vi "Meas Main.vi"(8 "error in":errorcluster, 11 "session in":variant) -> (0 "error out":errorcluster, 3 "session out":variant)   [LabVIEW 2013]
uses:
  Meas Session.ctl
  adc/ADC Session.ctl
  drivers/niScope/niScope Session.ctl
  drivers/niScope/niScope Virtual Channel Config.ctl
  drivers/niScope/niScope Virtual Channel Mode.ctl
  drivers/niScope/niScope Virtual Channel Input Z.ctl
  drivers/niScope/niScope Virtual Channel Coupling.ctl
  drivers/niScope/niScope Type.ctl
  drivers/niScope/niScope Digitizing Process Options.ctl
  drivers/niScope/niScope Data Packet.ctl
  drivers/niScope/niScope Trigger Setup.ctl
  <instrlib>/niScope/Controls/niScope trigger coupling.ctl
  <instrlib>/niScope/Controls/niScope trigger slope.ctl
  drivers/DMM/3458A Digitizer Session.ctl
  drivers/DMM/3458A Virtual Channel Config.ctl
  drivers/Counter/Counter Session.ctl
  drivers/Counter/Counter Type.ctl
  drivers/AWG/AWG Session.ctl
  drivers/AWG/AWG Type.ctl
  drivers/DMM/3458A Sync Mode.ctl
  drivers/DMM/3458A Idn Mode.ctl
  drivers/DMM/3458A Digitizing Low Levels/Configure/Sampling Mode.ctl
  drivers/DMM/3458A Digitizing Process Options.ctl
  drivers/DMM/3458A Data Packet.ctl
  drivers/DMM/3458A Aux Record Data.ctl
  drivers/DMM/3458A Digitizing Low Levels/Configure/Level Setup.ctl
  drivers/DMM/3458A Digitizing Low Levels/Configure/First Sample Trigger.ctl
  drivers/dsdll/DSDLL Session.ctl
  drivers/dsdll/dsdll.lvlibp/dsdll_instance.ctl
  drivers/dsdll/dsdll.lvlibp/dsdll_device_record.ctl
  drivers/dsdll/DSDLL Process Config.ctl
  drivers/dsdll/DSDLL Data Packet.ctl
  adc/ADC Type.ctl
  drivers/simulated_adc/SimAdc Config.ctl
  drivers/simulated_adc/SimAdc Channel Cfg.ctl
  adc/ADC On Close Action.ctl
  Meas Sequence Item.ctl
  Meas Sampling Configuration.ctl
  adc/ADC Trig Config.ctl
  adc/ADC Trig Mode Source.ctl
  adc/ADC Trig Coupling.ctl
  adc/ADC Trig Slope.ctl
  processing/QWTB/Meas Proc QWTB Algorithm Parameter Data.ctl
  Meas Sequence Configuration.ctl
  Meas Range Mode.ctl
  Meas Sampling Rate Mode.ctl
  octave/golpi/mpc/golpi_session_ref.ctl
  processing/Meas Process Config.ctl
  processing/Meas Process Mode.ctl
  processing/Meas Process Raw Config.ctl
  processing/Meas Process Raw Result Mode.ctl
  processing/QWTB/Meas Proc QWTB Setup.ctl
  processing/QWTB/Meas Proc QWTB Uncertainty Mode.ctl
  processing/QWTB/Meas Proc QWTB Multicore Setup.ctl
  processing/QWTB/Meas Proc QWTB Multicore Type.ctl
  Corrections/Corr Setup.ctl
  Corrections/Corr Tranducer Item.ctl
  Corrections/Corr Digitizers.ctl
  Assist/Assist Panel Setup.ctl
  varilib/SGUI Assign Multiple Strings With Tags By Label.vi
  drivers/niScope/niScope Virtual Digitizer.lvlib
  drivers/DMM/3458A Virtual Digitizer.lvlib
  drivers/Counter/Counter.lvlib
  drivers/AWG/AWG.lvlib
  drivers/DMM/3458A Digitizing Low Levels/3458A Digitizing Low Levels.lvlib
  varilib/varilib.lvlib
  drivers/dsdll/DSDLL Virtual Digitizer.lvlib
  drivers/dsdll/dsdll.lvlibp
  octave/golpi/mpc/GOLPI Multi Process.lvlib
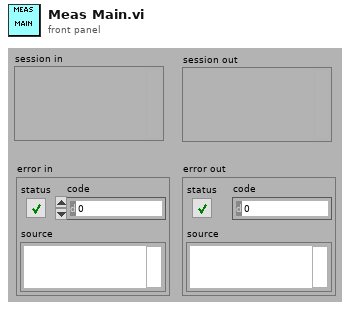
[diagram p1: front panel]
types:
  T1 = typedef "Meas Session.ctl" = cluster{"adc":T2, "sequence":T35[], "sequence setup":T42, "golpi":T45, "processing setup":T46, "corrections":T54, "assist cfg":T57}
  T2 = typedef "ADC Session.ctl" = cluster{"niScope":T3, "3458A":T13, "dsdll":T27, "type":T31, "channel idn str":string[], "aux instr idn str":string[], "modified?":bool, "simadc":T32, "force rst?":bool, "exit mode":T34, "exit dly":dbl, "exit tmr":timestamp, "busy?":bool, "accessed?":bool}
  T3 = typedef "niScope Virtual Digitizer.lvlib/niScope Session.ctl" = cluster{"channel cfg":T4[], "sessions":refnum<k20>[], "multi cards":bool, "channels":i32, "type":T8, "memory [B/chn]":i32, "ext. clock [Hz]":dbl, "samples count":i64, "use streaming":bool, "proc setup":T9, "sample width [B]":i32, "ranges [V]":dbl[], "trigger setup":T10, "fs [Hz]":dbl, "bitres [bit]":i32}
  T4 = typedef "niScope Virtual Digitizer.lvlib/niScope Virtual Channel Config.ctl" = cluster{"Address":refnum<k15>, "Channel":i32, "Mode":T5, "Input Z":T6, "Coupling":T7, "Range [Vpk]":dbl, "btn clr":bool, "btn up":bool, "btn down":bool}
  T5 = typedef "niScope Virtual Digitizer.lvlib/niScope Virtual Channel Mode.ctl" = enum16{"Single ended", "Unbal. differential", "Differential"}
  T6 = typedef "niScope Virtual Digitizer.lvlib/niScope Virtual Channel Input Z.ctl" = enum16{"1 MOhm", "50 Ohm"}
  T7 = typedef "niScope Virtual Digitizer.lvlib/niScope Virtual Channel Coupling.ctl" = enum16{"AC", "DC", "GND"}
  T8 = typedef "niScope Virtual Digitizer.lvlib/niScope Type.ctl" = enum16{"n/a", "5922"}
  T9 = typedef "niScope Virtual Digitizer.lvlib/niScope Digitizing Process Options.ctl" = cluster{"packet size [smpl]":i64, "current timeout [s]":dbl, "blk2blk timeout [s]":dbl, "event time":timestamp, "temp sampl T [s]":dbl, "data queue":refnum<queue>, "stop notifier":refnum<notifier>, "proc ref":refnum<vi>}
  T10 = typedef "niScope Virtual Digitizer.lvlib/niScope Trigger Setup.ctl" = cluster{"coupling":T11, "level [V]":dbl, "slope":T12, "mode":enum16{"Immediate", "External", "Level"}}
  T11 = typedef "niScope trigger coupling.ctl" = u16
  T12 = typedef "niScope trigger slope.ctl" = i32
  T13 = typedef "3458A Virtual Digitizer.lvlib/3458A Digitizer Session.ctl" = cluster{"channels":T14[], "sync unit":T15, "awg unit":T17, "sync mode":T19, "streaming mode":bool, "idn mode":T20, "sampling mode":T21, "Ts [s]":dbl, "sample memory [B]":i32, "proc setup":T22, "sample size [B]":i32, "sample count":i32, "aux data":T24, "ranges [V]":dbl[], "aperture [s]":dbl, "LEVEL trigger":T25, "trigger mode":T26, "measure temp.?":bool, "disp mesages":string[], "shared bus?":bool, "disable display?":bool}
  T14 = typedef "3458A Virtual Digitizer.lvlib/3458A Virtual Channel Config.ctl" = cluster{"VISA":refnum<visa-resource-name>, "Range [Vpk]":dbl, "btn clr":bool, "btn up":bool, "btn down":bool}
  T15 = typedef "Counter.lvlib/Counter Session.ctl" = cluster{"VISA":refnum<visa-resource-name>, "type":T16}
  T16 = typedef "Counter.lvlib/Counter Type.ctl" = enum16{"Picotest U6200A", "dummy"}
  T17 = typedef "AWG.lvlib/AWG Session.ctl" = cluster{"type":T18, "VISA":refnum<visa-resource-name>, "enable 10MHz ref":bool}
  T18 = typedef "AWG.lvlib/AWG Type.ctl" = enum16{"Agilent 331xxA to 332xxA", "Agilent 335xxA to 336xxA", "dummy"}
  T19 = typedef "3458A Virtual Digitizer.lvlib/3458A Sync Mode.ctl" = enum16{"MASTER-SLAVE, MASTER clocked by TIMER", "MASTER-SLAVE, MASTER clocked by AWG", "ALL clocked by AWG", "MASTER-SLAVE, ALL clocked by TIMER", "ALL clocked by AWG with DFLL"}
  T20 = typedef "3458A Virtual Digitizer.lvlib/3458A Idn Mode.ctl" = enum16{"Auto", "Sequential (chn A, chn B, ...)", "From calibration string"}
  T21 = typedef "3458A Virtual Digitizer.lvlib/3458A Digitizing Low Levels.lvlib/Sampling Mode.ctl" = enum16{"DCV", "DSDC", "DSAC"}
  T22 = typedef "3458A Virtual Digitizer.lvlib/3458A Digitizing Process Options.ctl" = cluster{"channel id":i32, "packet size [smpl]":i32, "current timeout [s]":dbl, "blk2blk timeout [s]":dbl, "event time":timestamp, "stop notifier":refnum<notifier>, "data queues":refnum<queue>[], "proc refs":refnum<vi>[], "bus semaphore":T23}
  T23 = typedef "Semaphore RefNum" = refnum<k1>
  T24 = typedef "3458A Virtual Digitizer.lvlib/3458A Aux Record Data.ctl" = cluster{"channel id":i32, "valid?":bool[], "gain [V]":dbl[], "timestamp [s]":dbl[], "Ts [s]":dbl, "abs timestamp":timestamp, "t [deg C]":dbl[]}
  T25 = typedef "3458A Virtual Digitizer.lvlib/3458A Digitizing Low Levels.lvlib/Level Setup.ctl" = cluster{"edge":enum16{"POS", "NEG"}, "level [V]":dbl, "coupling":enum16{"DC", "AC"}}
  T26 = typedef "3458A Virtual Digitizer.lvlib/3458A Digitizing Low Levels.lvlib/First Sample Trigger.ctl" = enum16{"AUTO", "EXT", "SYN", "SGL", "HOLD", "LEVEL"}
  T27 = typedef "DSDLL Virtual Digitizer.lvlib/DSDLL Session.ctl" = cluster{"dsdll":T28, "channels":i32, "device id":i32, "channel idns":string[], "proc setup":T30, "samples count":i32, "fs [Hz]":dbl}
  T28 = typedef "dsdll.lvlibp/dsdll_instance.ctl" = cluster{"dsdll path":path, "dsdll handle":u8[], "output devices":T29[], "capture devices":T29[]}
  T29 = typedef "dsdll.lvlibp/dsdll_device_record.ctl" = cluster{"guid":u8[], "name":string}
  T30 = typedef "DSDLL Virtual Digitizer.lvlib/DSDLL Process Config.ctl" = cluster{"packet size [smpl]":i32, "current timeout [s]":dbl, "blk2blk timeout [s]":dbl, "event time":timestamp, "data queue":refnum<queue>, "stop notifier":refnum<notifier>, "proc ref":refnum<vi>}
  T31 = typedef "ADC Type.ctl" = enum16{"niScope", "3458A", "DirectSound DLL", "dummy"}
  T32 = typedef "SimAdc Config.ctl" = cluster{"channels":T33[], "range [V]":dbl, "Ts step [s]":dbl, "time [s]":dbl, "fs [Hz]":dbl, "count":i64, "smpl offset":i64, "set count":i64, "bit res":i32}
  T33 = typedef "SimAdc Channel Cfg.ctl" = cluster{"harmonics":dbl[][], "btn clear":bool, "noise":dbl, "fundamental [Hz]":dbl}
  T34 = typedef "ADC On Close Action.ctl" = enum16{"Immediate reset", "Delayed reset"}
  T35 = typedef "Meas Sequence Item.ctl" = cluster{"config":T36, "data file path":path, "header file path":path, "group id":i32, "average id":i32, "group done?":bool, "adc modified?":bool, "source modified?":bool, "progress [%]":dbl, "groups cnt":i32, "average cnt":i32, "data file relative path":string, "meas root path":path, "calculate?":bool}
  T36 = typedef "Meas Sampling Configuration.ctl" = cluster{"fs [Hz]":dbl, "count [smpl]":i64, "aperture [s]":dbl, "trigger":T37, "ranges [Vpk]":dbl[], "QWTB parameters":T41[]}
  T37 = typedef "ADC Trig Config.ctl" = cluster{"source":T38, "level [V]":dbl, "coupling":T39, "slope":T40}
  T38 = typedef "ADC Trig Mode Source.ctl" = enum16{"Immediate", "External", "Level"}
  T39 = typedef "ADC Trig Coupling.ctl" = enum16{"DC", "AC"}
  T40 = typedef "ADC Trig Slope.ctl" = enum16{"POS", "NEG"}
  T41 = typedef "Meas Proc QWTB Algorithm Parameter Data.ctl" = cluster{"name":string, "numerics":dbl[], "strings":string[]}
  T42 = typedef "Meas Sequence Configuration.ctl" = cluster{"group setups":T36[], "average cycles":i32, "range mode":T43, "fs mode":T44, "rng even":dbl, "rng odd":dbl, "folder":path, "name base":string, "meas id":i32, "settle [s]":dbl}
  T43 = typedef "Meas Range Mode.ctl" = enum16{"Keep defaults", "Set All channels", "Set Odd and Even channels"}
  T44 = typedef "Meas Sampling Rate Mode.ctl" = enum16{"Frequency", "Period"}
  T45 = typedef "GOLPI Multi Process.lvlib/golpi_session_ref.ctl" = refnum<vi>
  T46 = typedef "Meas Process Config.ctl" = cluster{"mode":T47, "call after avgs?":bool, "calculate?":bool, "raw mode":T48, "QWTB":T50}
  T47 = typedef "Meas Process Mode.ctl" = enum16{"Raw", "QWTB"}
  T48 = typedef "Meas Process Raw Config.ctl" = cluster{"command":string, "result mode":T49, "res variable":string}
  T49 = typedef "Meas Process Raw Result Mode.ctl" = enum16{"Display console output (only Octave)", "Display string variable", "Display result file %respath%"}
  T50 = typedef "Meas Proc QWTB Setup.ctl" = cluster{"QWTB path":path, "alg filter path":string, "alg ids":string[], "alg parameters":string[], "parsed parameters":T41[], "selected alg id":string, "selected unc mode":T51, "qwtb mcc":i32, "qwtb timeout":i32, "qwtb covg":dbl, "qwtb ofs":i64, "qwtb lim data":i64, "multicore":T52, "unc once?":bool}
  T51 = typedef "Meas Proc QWTB Uncertainty Mode.ctl" = enum16{"None", "GUF", "Monte Carlo"}
  T52 = typedef "Meas Proc QWTB Multicore Setup.ctl" = cluster{"jobs folder":path, "cores":i32, "max jobs":i32, "mode":T53}
  T53 = typedef "Meas Proc QWTB Multicore Type.ctl" = enum16{"Singlecore", "Multicore", "Multistation"}
  T54 = typedef "Corr Setup.ctl" = cluster{"transducers":cluster{"channels":T55[], "last path":path}, "digitizer":T56}
  T55 = typedef "Corr Tranducer Item.ctl" = cluster{"Path":path, "Ratio:":string, "Name:":string, "btn rem":bool, "btn up":bool, "btn down":bool, "s.n.:":string, "btn open":bool, "ratio o/i":dbl, "chn hi":u16, "chn lo":u16, "Phase index":i32}
  T56 = typedef "Corr Digitizers.ctl" = cluster{"last path":path, "channel paths":path[], "channel idns":string[], "correction name":string, "channel names":string[], "folders to copy":path[], "channel valid":bool[], "correction path":path, "correction rel path":string, "rel folders to copy":string[]}
  T57 = typedef "Assist Panel Setup.ctl" = cluster{"P":i32, "Q":i32, "rel shift":dbl, "ref freq":dbl, "min fs":dbl, "max fs tol":dbl, "min int":dbl, "max int":dbl, "max err":dbl, "max timeout":dbl}
  T58 = typedef "GOLPI Multi Process.lvlib/golpi_session.ctl" = cluster{"GOLPI ref":T59, "idn str":string, "octave path":path, "work path":path, "start timeout [ms]":u32, "clr cache":bool, "console":bool, "binary":bool, "semaphore":T23, "initial command":string, "exit command":string, "matlab":bool}
  T59 = typedef "GOLPI Library.lvlibp/GOLPI reference Type Def.ctl" = cluster{"pipe handle":T60, "fast read timeout [ms]":u32, "fast read settle time [ms]":u32, "fast read to multiple [ms]":u32, "max elements per input line":u32, "slow read timeout [ms]":u32, "stdin double format specifier":string, "max elements per stdout output column":u32, "console mode bitstream":bool, "bitstream first read timeout [ms]":u32, "bitstream read timeout [ms]":u32, "struct transfer possible":bool, "matlab mode":bool}
  T60 = typedef "GOLPI Library.lvlibp/LV Process library.lvlib/Pipe Handle.ctl" = cluster{"lv_proc.dll file path":path, "process instance handle":u32[], "debug mode":bool, "debug data":cluster{"time":timestamp, "stdin":bool, "data":string}[]}
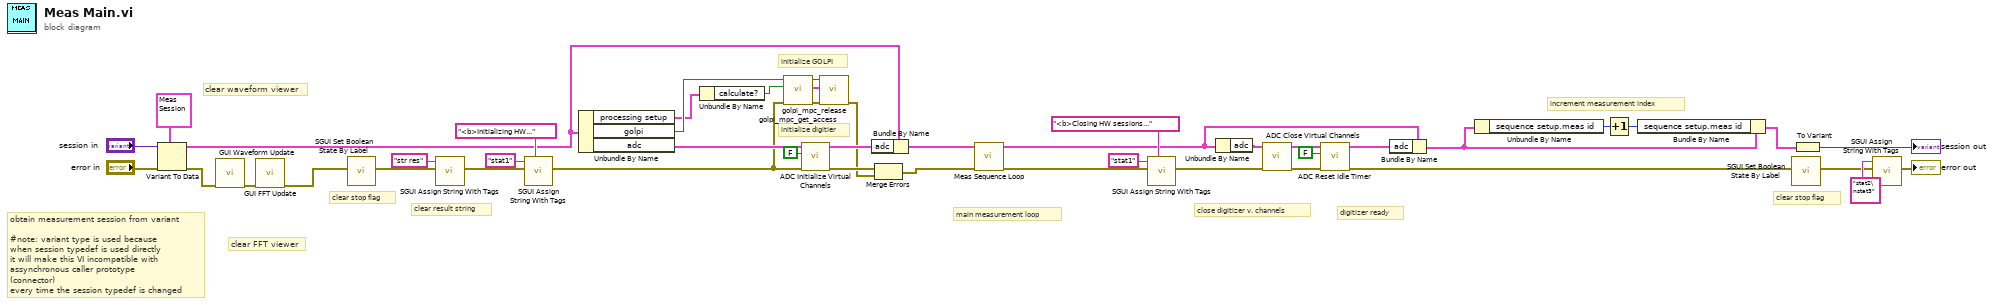
[diagram p0: block diagram]
diagram:
  # "clear FFT viewer"
  # "main measurement loop"
  # "digitizer ready"
  # "close digitizer v. channels"
  # "increment measurement index"
  # "clear waveform viewer"
  # "clear result string"
  # "initialize GOLPI"
  # "initialize digitier"
  # "clear stop flag"
  # "clear stop flag"
  # "obtain measurement session from variant\n\n#note: variant type is used because\nwhen session typedef is used directly \nit will make this VI incompatible with \nassynchronous caller prototype (connector)\nevery time the session typedef is changed"
  n1 = Variant To Data(error in="error in", type=T1 {"adc"={"niScope"={"channel cfg"=[], "sessions"=[], "multi cards"=FALSE, "channels"=0, "type"=enum."n/a", "memory [B/chn]"=0, "ext. clock [Hz]"=0.0, "samples count"=0, "use streaming"=FALSE, "proc setup"={"packet size [smpl]"=0, "current timeout [s]"=0.0, "blk2blk timeout [s]"=0.0, "event time"=timestamp(0 s since 1904-01-01), "temp sampl T [s]"=0.0, "data queue"=refnum, "stop notifier"=refnum, "proc ref"=refnum}, "sample width [B]"=0, "ranges [V]"=[], "trigger setup"={"coupling"=0, "level [V]"=0.0, "slope"=0, "mode"=enum."Immediate"}, "fs [Hz]"=0.0, "bitres [bit]"=0}, "3458A"={"channels"=[], "sync unit"={"VISA"="", "type"=enum."Picotest U6200A"}, "awg unit"={"type"=enum."Agilent 331xxA to 332xxA", "VISA"="", "enable 10MHz ref"=FALSE}, "sync mode"=enum."MASTER-SLAVE, MASTER clocked by TIMER", "streaming mode"=FALSE, "idn mode"=enum."Auto", "sampling mode"=enum."DCV", "Ts [s]"=0.0, "sample memory [B]"=0, "proc setup"={"channel id"=0, "packet size [smpl]"=0, "current timeout [s]"=0.0, "blk2blk timeout [s]"=0.0, "event time"=timestamp(0 s since 1904-01-01), "stop notifier"=refnum, "data queues"=[], "proc refs"=[], "bus semaphore"=refnum}, "sample size [B]"=0, "sample count"=0, "aux data"={"channel id"=0, "valid?"=[], "gain [V]"=[], "timestamp [s]"=[], "Ts [s]"=0.0, "abs timestamp"=timestamp(0 s since 1904-01-01), "t [deg C]"=[]}, "ranges [V]"=[], "aperture [s]"=0.0, "LEVEL trigger"={"edge"=enum."POS", "level [V]"=0.0, "coupling"=enum."DC"}, "trigger mode"=enum."AUTO", "measure temp.?"=FALSE, "disp mesages"=[], "shared bus?"=FALSE, "disable display?"=FALSE}, "dsdll"={"dsdll"={"dsdll path"=path "", "dsdll handle"=[], "output devices"=[], "capture devices"=[]}, "channels"=0, "device id"=0, "channel idns"=[], "proc setup"={"packet size [smpl]"=0, "current timeout [s]"=0.0, "blk2blk timeout [s]"=0.0, "event time"=timestamp(0 s since 1904-01-01), "data queue"=refnum, "stop notifier"=refnum, "proc ref"=refnum}, "samples count"=0, "fs [Hz]"=0.0}, "type"=enum."niScope", "channel idn str"=[], "aux instr idn str"=[], "modified?"=FALSE, "simadc"={"channels"=[], "range [V]"=0.0, "Ts step [s]"=0.0, "time [s]"=0.0, "fs [Hz]"=0.0, "count"=0, "smpl offset"=0, "set count"=0, "bit res"=0}, "force rst?"=FALSE, "exit mode"=enum."Immediate reset", "exit dly"=0.0, "exit tmr"=timestamp(0 s since 1904-01-01), "busy?"=FALSE, "accessed?"=FALSE}, "sequence"=[], "sequence setup"={"group setups"=[], "average cycles"=0, "range mode"=enum."Keep defaults", "fs mode"=enum."Frequency", "rng even"=0.0, "rng odd"=0.0, "folder"=path "", "name base"="", "meas id"=0, "settle [s]"=0.0}, "golpi"=refnum, "processing setup"={"mode"=enum."Raw", "call after avgs?"=FALSE, "calculate?"=FALSE, "raw mode"={"command"="", "result mode"=enum."Display console output (only Octave)", "res variable"=""}, "QWTB"={"QWTB path"=path "", "alg filter path"="", "alg ids"=[], "alg parameters"=[], "parsed parameters"=[], "selected alg id"="", "selected unc mode"=enum."None", "qwtb mcc"=0, "qwtb timeout"=0, "qwtb covg"=0.0, "qwtb ofs"=0, "qwtb lim data"=0, "multicore"={"jobs folder"=path "", "cores"=0, "max jobs"=0, "mode"=enum."Singlecore"}, "unc once?"=FALSE}}, "corrections"={"transducers"={"channels"=[], "last path"=path ""}, "digitizer"={"last path"=path "", "channel paths"=[], "channel idns"=[], "correction name"="", "channel names"=[], "folders to copy"=[], "channel valid"=[], "correction path"=path "", "correction rel path"="", "rel folders to copy"=[]}}, "assist cfg"={"P"=0, "Q"=0, "rel shift"=0.0, "ref freq"=0.0, "min fs"=0.0, "max fs tol"=0.0, "min int"=0.0, "max int"=0.0, "max err"=0.0, "max timeout"=0.0}} ("session in"), Variant="session in") -> (data=w25:T1, error out=w12:errorcluster)
  n2 = call "GUI Waveform Update.vi"("error in"=w12) -> ("error out"=w2:errorcluster)  [unwired: 10 in]
  n3 = call "GUI FFT Update.vi"("error in"=w2) -> ("error out"=w1:errorcluster)  [unwired: 10 in]
  n4 = call "SGUI Set Boolean State By Label.vi"("error in"=w1) -> ("error out"=w15:errorcluster)  [unwired: 9 in, 1 out]
  n5 = call-poly "SGUI Assign String With Tags.vi"("error in"=w15, "label(s) (empty)"="str res") -> ("error out"=w14:errorcluster)  [unwired: 8 in, 1 out]
  n6 = call-poly "SGUI Assign String With Tags.vi"("error in"=w14, "label(s) (empty)"="stat1", "string (empty)"="<b>Initializing HW...") -> ("error out"=w16:errorcluster)  [unwired: 7 in, 1 out]
  n7 = Unbundle By Name(w25) -> ("processing setup"=w21:T46, "golpi"=w22:T45, "adc"=w45:T2)
  n8 = Unbundle By Name(w21) -> ("calculate?"=w20:bool)
  n9 = call "golpi_mpc_get_access.vi"("error in"=w16, "allow octave start (true)"=w20, "golpi session ref"=w22) -> ("error out"=w24:errorcluster, "golpi session out"=w23:T58, "golpi session ref out (copy)"=w26:T45)  [unwired: 3 in, 3 out]
  n10 = call "ADC Initialize Virtual Channels.vi"("error in"=w16, "Reset? (False)"=FALSE, "adc session in"=w45) -> ("error out"=w19:errorcluster, "adc session out"=w40:T2)  [unwired: 4 in, 3 out]
  n11 = call "golpi_mpc_release.vi"("error in"=w24, "golpi ref or golpi session in"=w23, "golpi session ref"=w26) -> ("error out"=w18:errorcluster)  [unwired: 7 in, 1 out]
  n12 = Bundle By Name(cluster=w25, "adc"=w40) -> (w38:T1)
  n13 = Merge Errors(w19, w18) -> (w17:errorcluster)
  n14 = call "Meas Sequence Loop.vi"("error in"=w17, "meas session in"=w38) -> ("error out"=w33:errorcluster, "meas session out"=w32:T1)  [unwired: 8 in]
  n15 = call-poly "SGUI Assign String With Tags.vi"("error in"=w33, "label(s) (empty)"="stat1", "string (empty)"="<b>Closing HW sessions...") -> ("error out"=w31:errorcluster)  [unwired: 7 in, 1 out]
  n16 = Unbundle By Name(w32) -> ("adc"=w39:T2)
  n17 = call "ADC Close Virtual Channels.vi"("error in"=w31, "adc session in"=w39) -> ("error out"=w7:errorcluster, "adc session out"=w6:T2)  [unwired: 8 in]
  n18 = call "ADC Reset Idle Timer.vi"("error in"=w7, "set busy (False)"=FALSE, "adc session in"=w6) -> ("error out"=w4:errorcluster, "adc session out"=w5:T2)  [unwired: 7 in]
  n19 = Bundle By Name(cluster=w32, "adc"=w5) -> (w10:T1)
  n20 = Unbundle By Name(w10) -> ("sequence setup.meas id"=w11:i32)
  n21 = Increment(x=w11) -> (x+1=w9:i32)
  n22 = Bundle By Name(cluster=w10, "sequence setup.meas id"=w9) -> (w8:T1)
  n23 = call "SGUI Set Boolean State By Label.vi"("error in"=w4) -> ("error out"=w29:errorcluster)  [unwired: 9 in, 1 out]
  n24 = To Variant(anything=w8) -> (Variant=→"session out":variant)
  n25 = call-poly "SGUI Assign String With Tags.vi"("error in"=w29, "label(s) (empty)"="stat2\nstat3") -> ("error out"=→"error out":errorcluster)  [unwired: 8 in, 1 out]
